vi "Run In Test SAA.vi"(8 "error in (no error)":errorcluster, 10 "Model in":refnum<class "Model.lvclass">, 11 "Test Actuator State in":refnum<class "Test Actuator State.lvclass">) -> (0 "error out":errorcluster, 1 "Pass":bool, 2 "Model out":refnum<class "Model.lvclass">, 3 "Test Actuator State out":refnum<class "Test Actuator State.lvclass">)   [LabVIEW 2016, in "Test Actuator State.lvclass"]
uses:
  Test Actuator State.lvclass
  Model/Model/Model.lvclass
  <vilib>/Platform/TimedLoop/XDataNode/timing_clust.ctl
  <vilib>/Platform/TimedLoop/XDataNode/nitl_modes.ctl
  <vilib>/Platform/TimedLoop/XDataNode/wakeup.ctl
  Model/Model/Model.lvclass/Model.ctl
  Typedefs/ActuatorSetPoints.ctl
  <vilib>/platform/TimedLoop/XDataNode/XDataNode.xnode
  Typedefs/FAMT Typedefs.lvlib
  <vilib>/Platform/TimedLoop/XDataNode/XDNodeRunTimeDep.lvlib
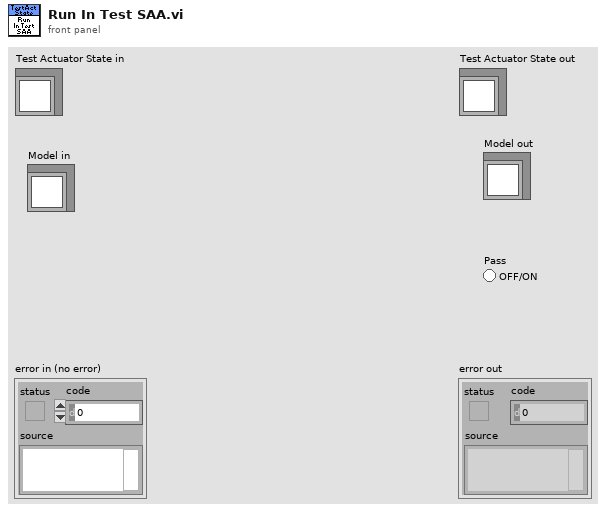
[diagram p1: front panel]
types:
  T1 = typedef "FAMT Typedefs.lvlib/RunInSettings.ctl" = cluster{"Hold Time (s)":dbl, "Iterations":i32}
  T2 = typedef "FAMT Typedefs.lvlib/FullForceScanSettings.ctl" = cluster{"Force Tolerance (N)":dbl, "DAA Force Set Points":T3[], "Process Time (s)":dbl, "Sample Time (s)":dbl, "SAA Force Set Points":T3[]}
  T3 = typedef "FAMT Typedefs.lvlib/ForcePair.ctl" = cluster{"Axial Force":dbl, "Lateral Force":dbl}
  T4 = typedef "XDNodeRunTimeDep.lvlib/timing_clust.ctl" = cluster{"Expected End [f-1]":u64, "Actual End [f-1]":u64, "Finished Late? [f-1]":bool, "Expected End [i-1]":u64, "Actual End [i-1]":u64, "Finished Late? [i-1]":bool, "Expected Start [i]":u64, "Actual Start [i]":u64, "Expected Start [f]":u64, "Actual Start [f]":u64, "Source Name":string, "Structure Name":string, "Period":i64, "Deadline":i64, "Offset":i64, "Start":i64, "Priority":i32, "Timeout":i32, "Mode":T5, "Wakeup Reason":T6, "Error":errorcluster, "Source Type":string, "Secondary Source Type":string, "Global End Time":u64, "Global Start Time":u64, "Frame Duration":u64, "Iteration Duration":u64, "Assigned CPU":i32, "I/O Scan Engine Mode":u32}
  T5 = typedef "XDNodeRunTimeDep.lvlib/nitl_modes.ctl" = enum32{"No Change", "Process missed periods, maintain original phase", "Discard missed periods, maintain original phase", "Process missed periods, ignore original phase", "Discard missed periods, ignore original phase"}
  T6 = typedef "XDNodeRunTimeDep.lvlib/wakeup.ctl" = enum32{"Normal", "Aborted", "Asynchronous wakeup", "Timing source error", "Timed loop error", "Timeout"}
  T7 = typedef "FAMT Typedefs.lvlib/ActuatorSetPoints.ctl" = cluster{"Axial Force":dbl, "Lateral Force":dbl, "FC1 Force":dbl, "FC2 Force":dbl}
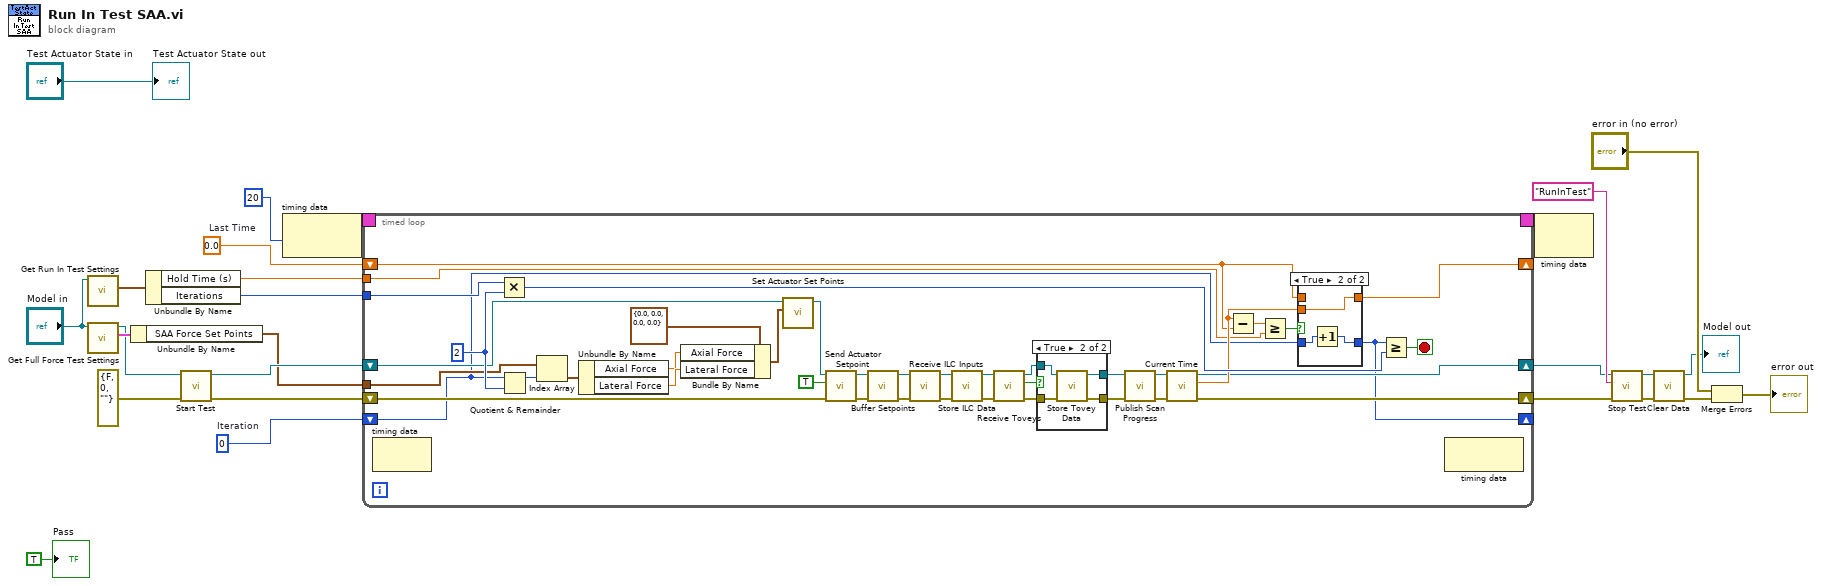
[diagram p0: block diagram]
diagram:
  w3 = 0  # Iteration
  w9 = 0.0  # Last Time
  n1 = call "Get Run In Test Settings.vi"("Model in"="Model in") -> ("Run In Test Settings"=w19:T1)  [unwired: 9 in, 1 out]
  n2 = call "Get Full Force Test Settings.vi"("Model in"="Model in") -> ("Full Force Test Settings"=w23:T2, "Model out"=w18:refnum<class "Model.lvclass">)  [unwired: 9 in]
  n3 = Unbundle By Name(w23) -> ("SAA Force Set Points"=w5:T3[])
  n4 = Unbundle By Name(w19) -> ("Hold Time (s)"=w8:dbl, "Iterations"=w7:i32)
  n5 = call "Start Test.vi"("error in (no error)"=errorcluster {"status"=FALSE, "code"=0, "source"=""} ("error out"), "Model in"=w18) -> ("error out"=w4:errorcluster, "Model out"=w6:refnum<class "Model.lvclass">)  [unwired: 8 in]
  n6 = node-c288(i64 20 ("Period")) -> (w12:T4)
  n7 = timed-loop {
    timing: w12 -> [_]
    timing-out: [_] -> w11
    shift-right: [w31] -> _
    shift-left: w9 -> [w38]
    tunnel: w8 -> [w37]
    tunnel: w7 -> [w36]
    shift-right: [w30] -> w2
    shift-left: w6 -> [w35]
    tunnel: w5 -> [w34]
    shift-right: [w29] -> w1
    shift-left: w4 -> [w33]
    shift-right: [w28] -> _
    shift-left: w3 -> [w32]
    stop <- w27 stop-if-true
    w64 = 2 ("y")
    n8 = node-c288() -> ()  [unwired: 1 in, 1 out]
    n9 = Multiply(x=w36, y=w64) -> (x*y=w65:i32)
    n10 = Quotient & Remainder(x=w32, y=w64) -> (x-y*floor(x/y)=w63:i32)  [unwired: 1 out]
    n11 = Index Array(array=w34, index=w63) -> (element=w54:T3)
    n12 = Unbundle By Name(w54) -> ("Axial Force"=w56:dbl, "Lateral Force"=w57:dbl)
    n13 = Bundle By Name(cluster=T7 {"Axial Force"=0.0, "Lateral Force"=0.0, "FC1 Force"=0.0, "FC2 Force"=0.0} ("Actuator Set Points"), "Axial Force"=w56, "Lateral Force"=w57) -> (w58:T7)
    n14 = call "Set Actuator Set Points.vi"("Actuator Set Points"=w58, "Model in"=w35) -> ("Model out"=w59:refnum<class "Model.lvclass">)  [unwired: 9 in]
    n15 = call "Send Actuator Setpoint.vi"("error in (no error)"=w33, "SlewFlag"=TRUE, "Model in"=w59) -> ("error out"=w52:errorcluster, "Model out"=w50:refnum<class "Model.lvclass">)  [unwired: 7 in]
    n16 = call "Buffer Setpoints.vi"("error in (no error)"=w52, "Model in"=w50) -> ("error out"=w53:errorcluster, "Model out"=w51:refnum<class "Model.lvclass">)  [unwired: 8 in]
    n17 = call "Receive ILC Inputs.vi"("error in (no error)"=w53, "Model in"=w51) -> ("error out"=w49:errorcluster, "Model out"=w48:refnum<class "Model.lvclass">)  [unwired: 8 in]
    n18 = call "Store ILC Data.vi"("error in (no error)"=w49, "Model in"=w48) -> ("error out"=w40:errorcluster, "Model out"=w39:refnum<class "Model.lvclass">)  [unwired: 8 in]
    n19 = call "Receive Toveys.vi"("error in (no error)"=w40, "Model in"=w39) -> ("error out"=w42:errorcluster, "Data Received"=w43:bool, "Model out"=w41:refnum<class "Model.lvclass">)  [unwired: 7 in]
    n20 = case shown="True" w43 {
      tunnel: w41 -> [w73 w77]
      tunnel: w42 -> [w72 w76]
      tunnel: [w72 w75] -> w47
      tunnel: [w73 w74] -> w44
      frame False {
      }
      frame True {
        n21 = call "Store Tovey Data.vi"("error in (no error)"=w76, "Model in"=w77) -> ("error out"=w75:errorcluster, "Model out"=w74:refnum<class "Model.lvclass">)  [unwired: 8 in]
      }
    }
    n22 = call "Publish Scan Progress.vi"("error in (no error)"=w47, "Model in"=w44) -> ("error out"=w46:errorcluster, "Model out"=w45:refnum<class "Model.lvclass">)  [unwired: 8 in]
    n23 = call "Current Time.vi"("error in (no error)"=w46, "Model in"=w45) -> ("error out"=w29:errorcluster, "Time"=w62:dbl, "Model out"=w30:refnum<class "Model.lvclass">)  [unwired: 7 in]
    n24 = Subtract(x=w62, y=w38) -> (x-y=w60:dbl)
    n25 = Greater Or Equal?(x=w60, y=w37) -> (x >= y?=w61:bool)
    n26 = case shown="True" w61 {
      tunnel: w62 -> [_ w71]
      tunnel: w38 -> [w68 _]
      tunnel: [w68 w71] -> w31
      tunnel: w32 -> [w67 w70]
      tunnel: [w67 w69] -> w28
      frame False {
      }
      frame True {
        n27 = Increment(x=w70) -> (x+1=w69:i32)
      }
    }
    n28 = Greater Or Equal?(x=w28, y=w65) -> (x >= y?=w27:bool)
    n29 = node-c288() -> ()  [unwired: 1 in, 1 out]
  }
  n30 = node-c288(w11) -> ()  [unwired: 1 out]
  n31 = call "Stop Test.vi"("error in (no error)"=w1, "Test"="RunInTest", "Model in"=w2) -> ("error out"=w16:errorcluster, "Model out"=w17:refnum<class "Model.lvclass">)  [unwired: 7 in]
  n32 = call "Clear Data.vi"("error in (no error)"=w16, "Model in"=w17) -> ("error out"=w14:errorcluster, "Model out"=→"Model out":refnum<class "Model.lvclass">)  [unwired: 8 in]
  n33 = Merge Errors("error in (no error)", w14) -> (→"error out":errorcluster)
  "Test Actuator State out" <- "Test Actuator State in"
  "Pass" <- TRUE ("Pass")
